vi "Dashboard Main.vi"() -> ()   [LabVIEW 2018]
uses:
  <vilib>/Rock Robotics/WPI/Camera/WPI_CameraSettings Read MJPG.ctl
  <vilib>/Rock Robotics/WPI/Camera/WPI_CameraImageSize.ctl
  <vilib>/Utility/miscctls.llb/LVPointTypeDef.ctl
  <vilib>/Utility/miscctls.llb/LVBoundsTypeDef.ctl
  <vilib>/Rock Robotics/Network Tables/NT Read Number.vi
  <vilib>/Rock Robotics/Network Tables/NT Write String.vi
  <vilib>/Rock Robotics/Network Tables/NT Write Number.vi
  <vilib>/Rock Robotics/WPI/Dashboard/WPI_DashboardLogging Global.vi
  <vilib>/Rock Robotics/Network Tables/NT Read Variant.vi
panel:
  out "Camera Perf":string
  out "Right Camera Perf":cluster{"Bandwidth (Mbps)":dbl, "FPS":dbl}
  out "NT Connection":bool
  in  "Driver Configuration":enum16{"James", "Ryan"}(ring)
  in  "Camera Settings Right":T1={"Frame Rate"=30, "Compression"=30, "Size"=1, "DB Camera Config"=FALSE} {"Frame Rate" scale=1.0..30.0; "Compression" scale=100.0..-1.0; "Size" items=["640x480", "320x240", "160x120"]}
  in  "Camera Name Right":string(combo)="No Camera Selection"
  in  "TCP":refnum<k5>
  in  "Rec Mode":enum32{"Stop", "Record", "Playback"}(radio)
  out "Robot IP":string
  out "Image Message":string="Timeout in Camera Communications"
  in  "Dashboard Tab":T2(tab)
  out "Pressure":u8(slide) scale=0.0..140.0
  out "Time":dbl
  out "Camera Image Right":T3(plugin-control)
  in  "Camera Settings":T4={"fps"=30, "compression"=30, "Image Size"=enum."320x240", "Config Shown"=FALSE}
  out "Endgame?":bool
  out "Stilts":bool
  out "Rhino":bool
  out "Floating":bool
  out "Carriage":bool
  out "Cascade":bool
  out "Errors":string
  out "Drive Base":bool
  out "Postmatch Pressure Log":dbl(graph)
  out "Mode":T6(ring)=enum."Auto Disabled"
  out "IMU":dbl
  out "Picture":picture
  in  "Autonomous Selector":T7(ring)
  out "Picture 2":picture
  out "Tree":string(tree)
  # "HW"
  # "Robot Health"
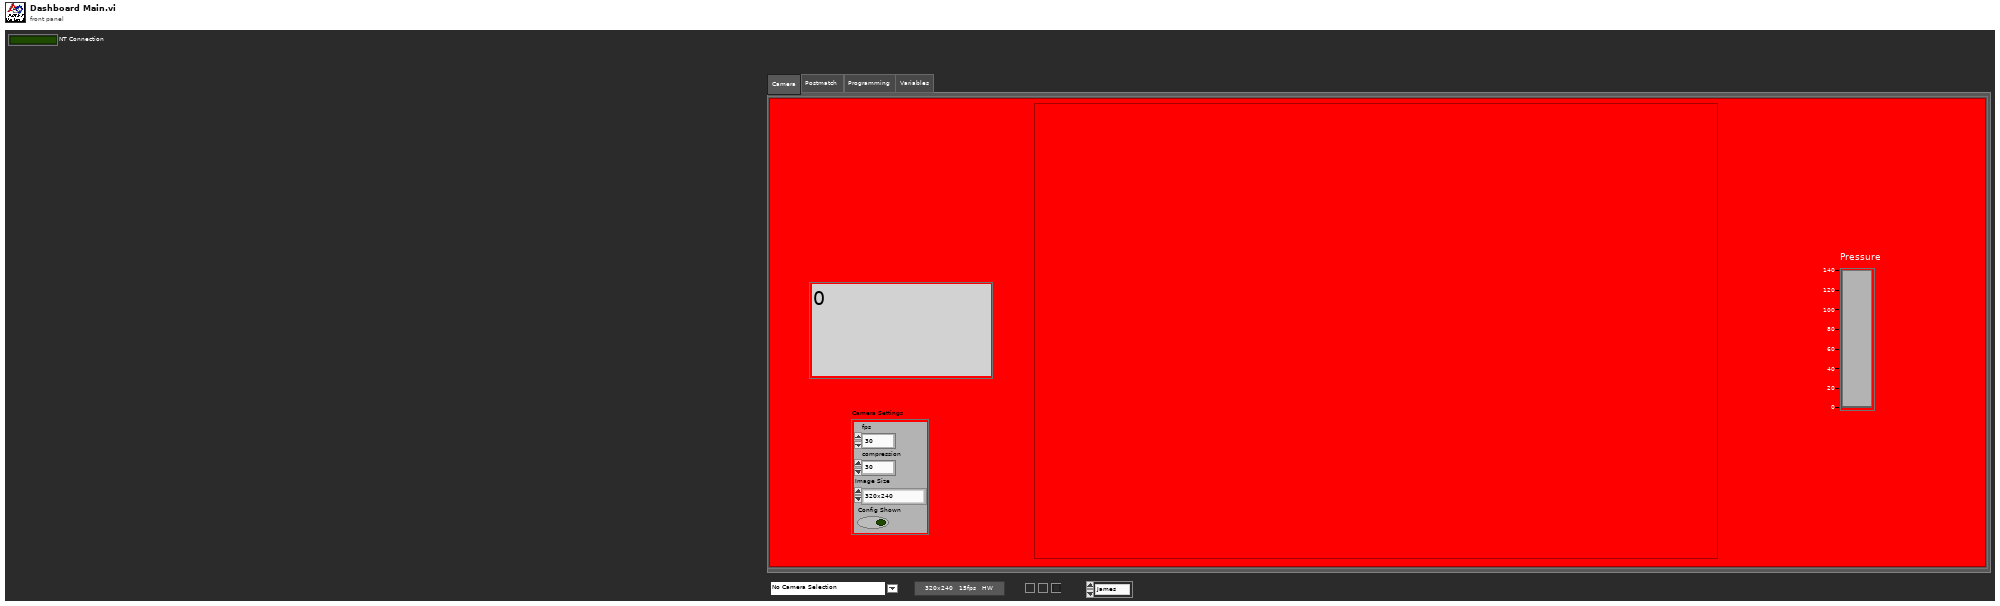
[diagram p1: front panel]
types:
  T1 = cluster{"Frame Rate":i32, "Compression":i32, "Size":u16, "DB Camera Config":bool}
  T2 = enum32{"Camera", "Postmatch", "Programming", "Variables"}
  T3 = typedef "IMAQ Image.ctl" = refnum<image>
  T4 = typedef "WPI_CameraSettings Read MJPG.ctl" = cluster{"fps":i32, "compression":i32, "Image Size":T5, "Config Shown":bool}
  T5 = typedef "WPI_CameraImageSize.ctl" = enum16{"640x480", "320x240", "160x120", "Custom"}
  T6 = enum8{"Tele-Op Disabled", "Tele-Op Enabled", "Auto Disabled", "Auto Enabled", "Test Disabled", "Test Enabled", "Disconnected", "No Code", "E-Stop"}
  T7 = enum16{"Teleop", "Double Rocket L", "Double Rocket R", "Side Cargo L", "Side Cargo R", "Double Front L", "Double Front R"}
  T8 = typedef "LVBoundsTypeDef.ctl" = cluster{"Width":u32, "Height":u32}
  T9 = typedef "LVPointTypeDef.ctl" = cluster{"Horizontal":i16, "Vertical":i16}
  T10 = cluster{"Save Path":path, "Interval (s)":dbl, "Keep":i32}
  T11 = enum32{"Drive", "Camera", "Basic", "Custom", "Test", "Commands", "Checklist", "Variables"}
  T12 = typedef "Image Type" = u32
  T13 = cluster{"IDs":cluster{"RPC field ID":u16, "Unique ID":u16}, "String":string}
  T14 = enum8{"Enabled", "Disabled", "Disabled and Grayed Out"}
  T15 = cluster{"Error Strings":string, "Disable Counts":cluster{u16, u16}, "Rail Faults":cluster{u16, u16, u16}, "Robot IP":string, "DB Mode":u8, "Event Info":cluster{"Name":string, "Type":u8, "Number":u16, "Replay":u8}}
  T16 = cluster{"Storage":cluster{"Disk Free":u64, "RAM Block":u32, "RAM free":u32}, "CPU Utilization":cluster{"CPU % ISR":sgl, "CPU % Time Crit":sgl, "CPU % Timed Str":sgl, "CPU % High":sgl, "CPU % Above":sgl, "CPU % Normal":sgl, "CPU % Low":sgl}, "CAN":cluster{"% Bus Utilization":sgl, "Bus Off Cnt":u32, "TX_FIFO Full Cnt":u32, "Receive Error Cnt":u8, "Transmit Error Cnt":u8}, "HID":cluster{"HID Outputs":u32, "Rumble Low":u16, "Rumble High":u16}[]}
  T17 = cluster{"Status bits":cluster{"Test Mode":bool, "Autonomous":bool, "Enabled":bool, "Code Start":bool, "Brownout":bool, "Reserved 2":bool, "Reserved 3":bool, "E-Stop":bool}, "Code Trace":cluster{"Disabled":bool, "TeleOp":bool, "Auto":bool, "Test":bool}, "Controller Type":enum16{"unknown", "cRIO", "roboRio"}, "Code?":enum16{"unknown", "noCode", "code"}, "Battery V":dbl}
  T18 = cluster{"Control Bits":cluster{"TestMode":bool, "Autonomous":bool, "Enabled":bool, "FMS Present":bool, bool, bool, bool, "E-Stop":bool}, "Team Station ":u8, "Countdown":sgl, "Joystick Values":cluster{"Axes":dbl[], "Buttons":bool[], "POVs":i16[]}[]}
  T19 = cluster{"Axes":dbl[], "Buttons":bool[], "POVs":i16[]}[]
  T20 = cluster{"Axes":dbl[], "Buttons":bool[], "POVs":i16[]}
  T21 = cluster{"Global Rectangle":i32[], "Contours":cluster{"Contour Type":u32, "ROI Type":u32, "Points":i32[]}[]}
  T22 = cluster{"Camera Name Right":string, string, "Saved DB Images Info":cluster{"Save Path":path, "Interval (s)":dbl, "Keep":i32}}
  T23 = cluster{"Operation":enum16{"Update", "Clear"}, "Color Box":u32}[]
  T24 = cluster{"Image Size":bool, "Image Type":bool, "Pixel Value":bool, "ROI Information":bool, "Zoom Factor":bool}
  T25 = cluster{"Shift":bool, "Ctrl":bool, "Alt":bool, "Cmd":bool, "Opt":bool}
  T26 = cluster{"Segment Name":string, "Type":enum16{"Accel Straight", "Const Straight", "Blend", "Circle"}, "Traj Pos Points":cluster{"x":dbl, "y":dbl, "th":dbl}[], "Traj Vel Points":cluster{"V":dbl, "th":dbl}[], "Accel Index":i32, "Decel Index":i32}[]
  T27 = cluster{"Index":i32, "Pt Test Results":enum16{"Miss", "Rect Hit", "Arrow Hit"}}
  T28 = cluster{"Points":cluster{"x":dbl, "y":dbl, "th":dbl}[], "Trajectory Data":cluster{"Segment Name":string, "Type":enum16{"Accel Straight", "Const Straight", "Blend", "Circle"}, "Traj Pos Points":cluster{"x":dbl, "y":dbl, "th":dbl}[], "Traj Vel Points":cluster{"V":dbl, "th":dbl}[], "Accel Index":i32, "Decel Index":i32}[]}
  T29 = cluster{"Points":cluster{"x":dbl, "y":dbl, "th":dbl}[], "Trajectory Data":cluster{"Segment Name":string, "Type":enum16{"Accel Straight", "Const Straight", "Blend", "Circle"}, "Traj Pos Points":cluster{"x":dbl, "y":dbl, "th":dbl}[], "Traj Vel Points":cluster{"V":dbl, "th":dbl}[], "Accel Index":i32, "Decel Index":i32}[]}[]
  T30 = cluster{"Horizontal":dbl, "Vertical":dbl, "th":dbl}
  T31 = typedef "imagedata.ctl" = cluster{"image type":i32, "image depth":i32, "image":u8[], "mask":u8[], "colors":u32[], "Rectangle":cluster{"left":i16, "top":i16, "right":i16, "bottom":i16}}
  T32 = typedef "LVRectTypeDef.ctl" = cluster{"Left":i16, "Top":i16, "Right":i16, "Bottom":i16}
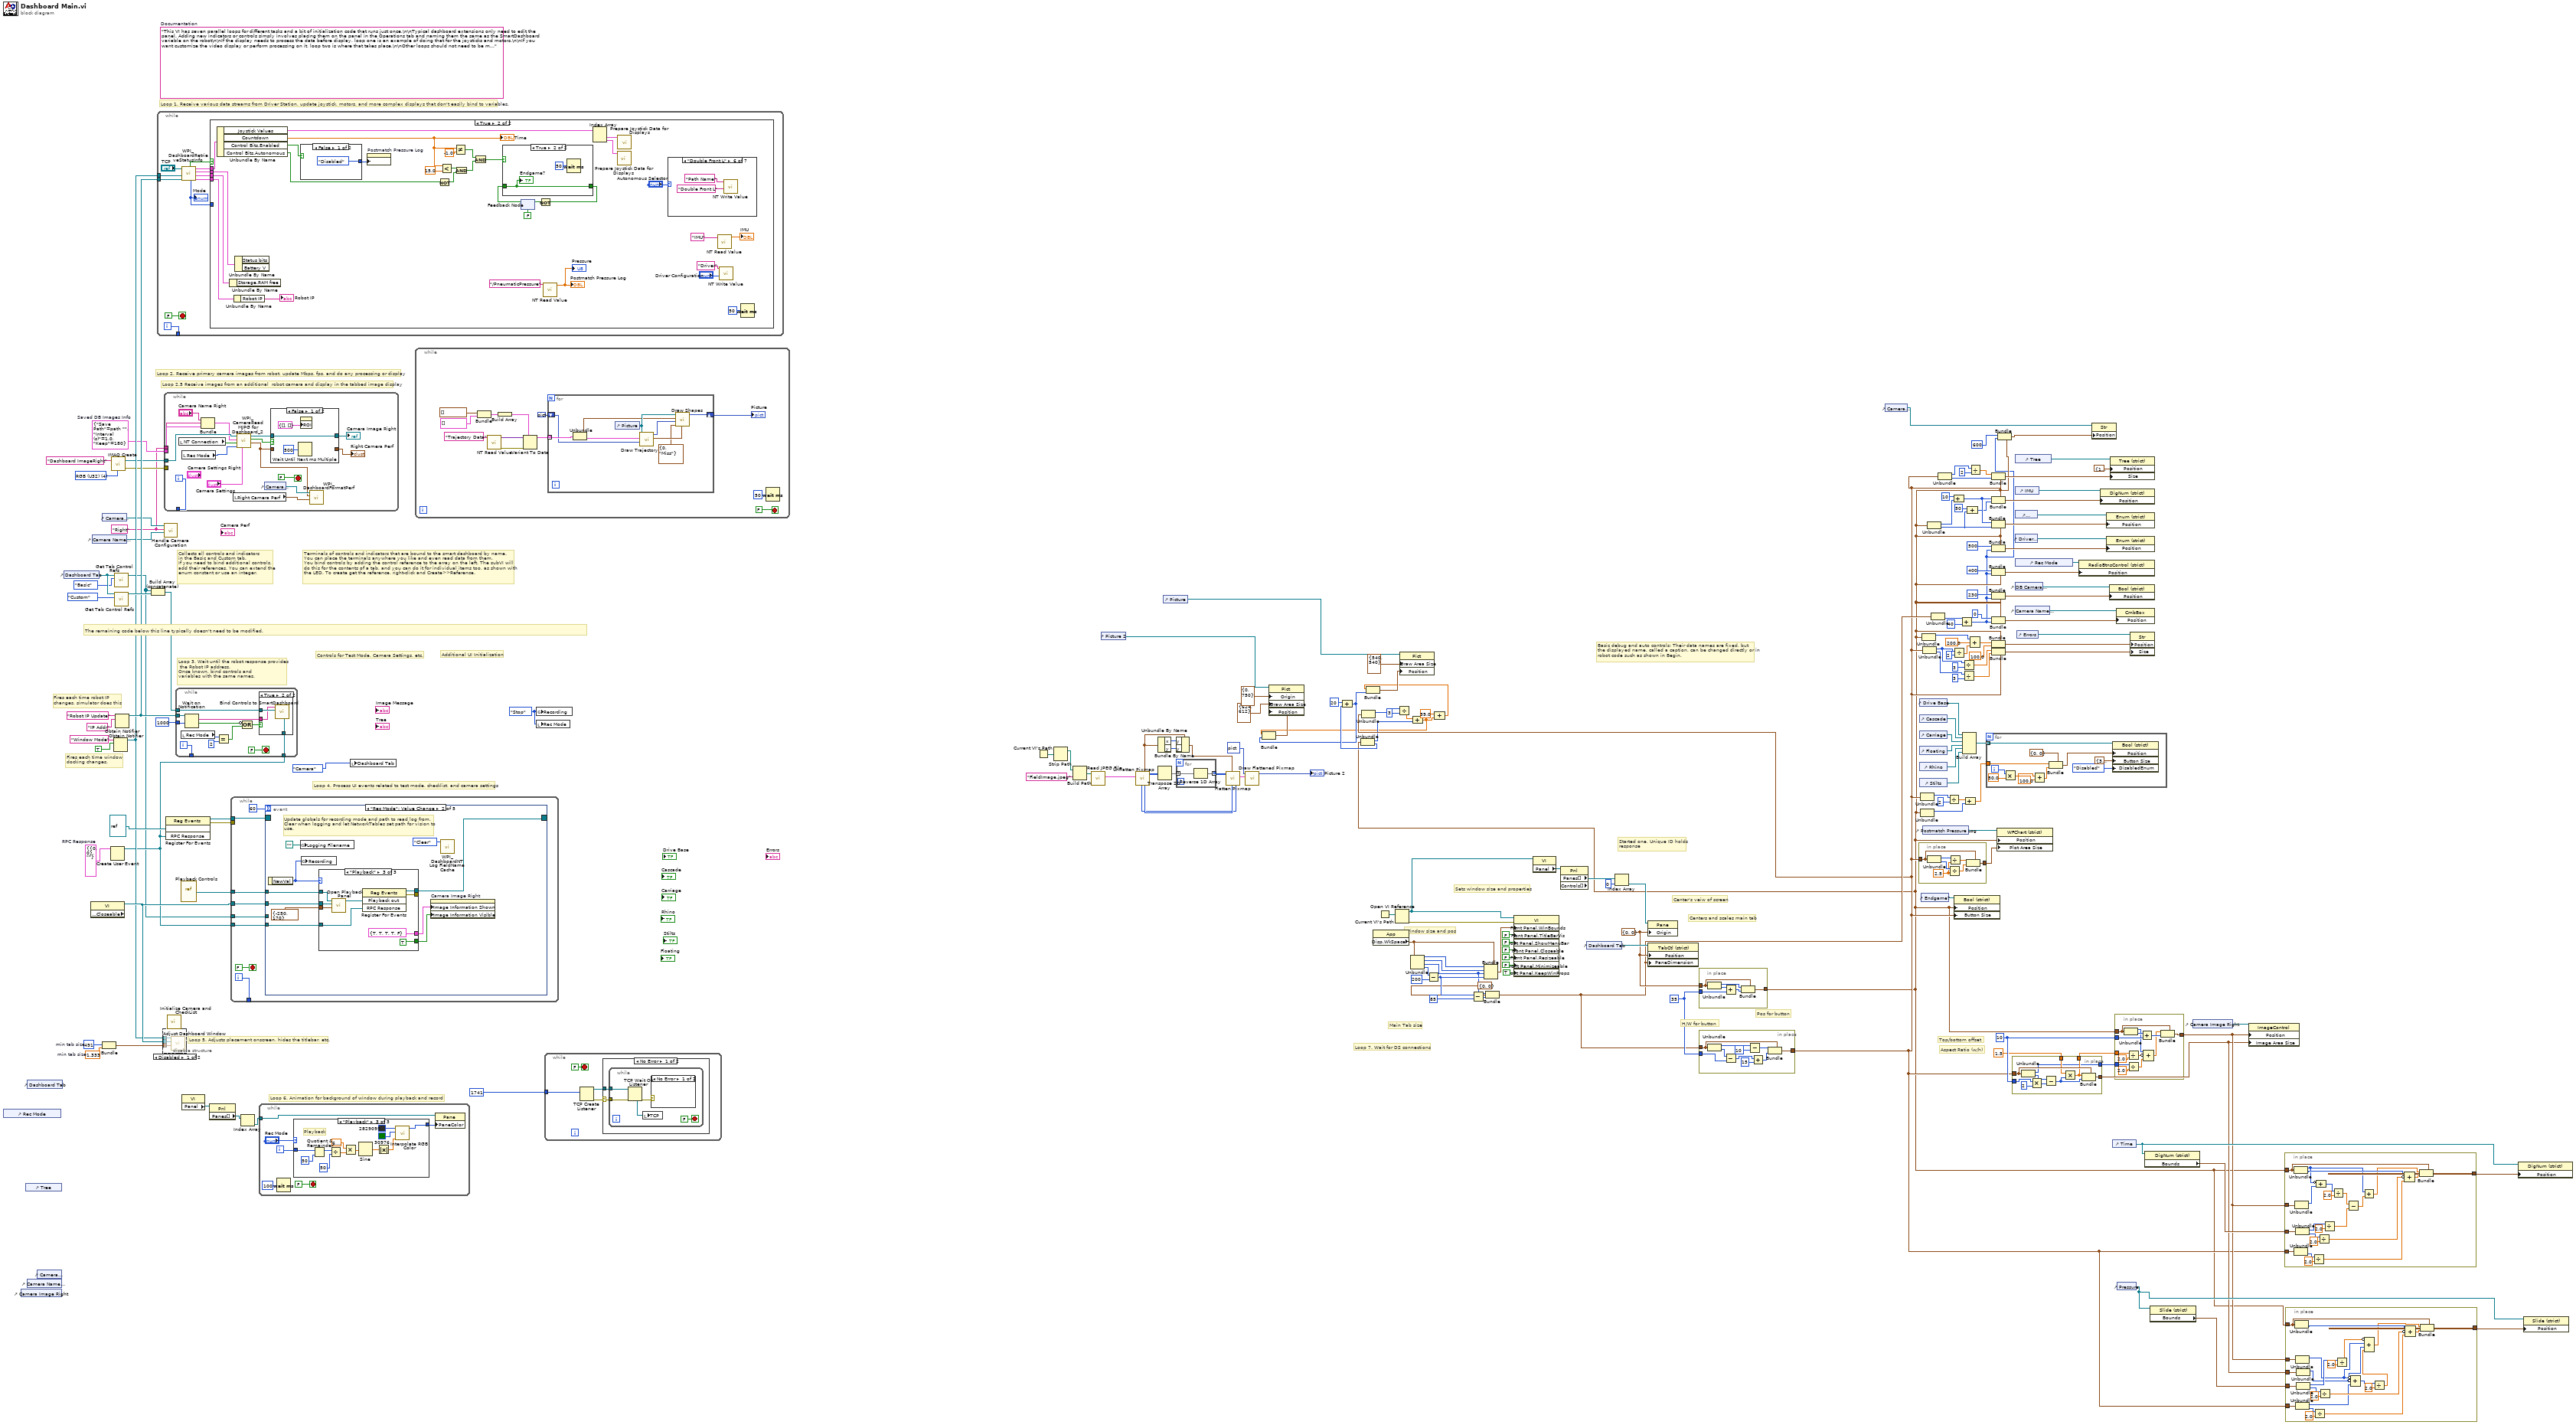
[diagram p0: block diagram]
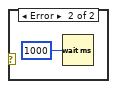
[diagram p4: hidden frame]
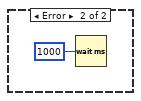
[diagram p5: hidden frame]
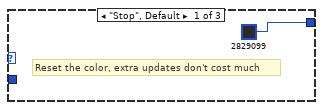
[diagram p6: hidden frame]
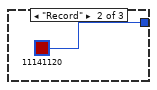
[diagram p7: hidden frame]
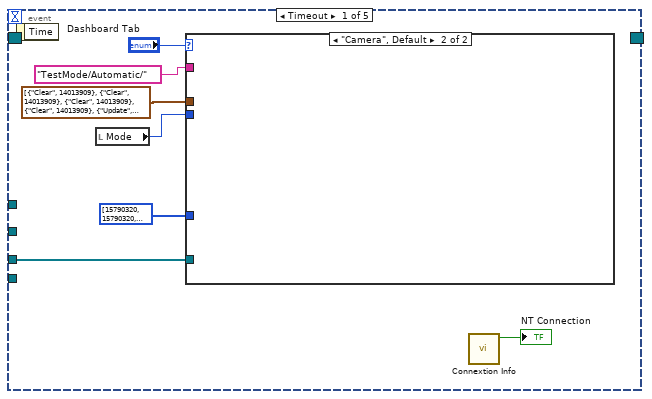
[diagram p9: hidden frame]
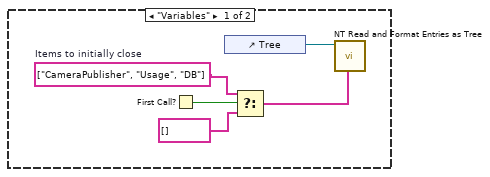
[diagram p10: hidden frame]
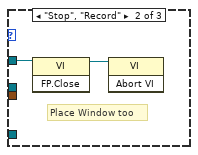
[diagram p12: hidden frame]
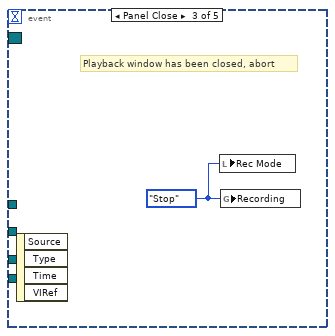
[diagram p13: hidden frame]
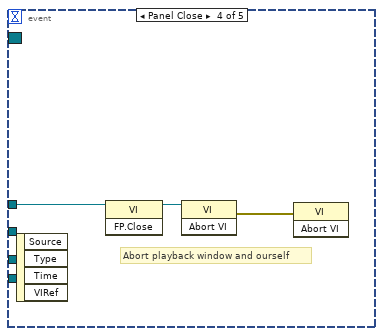
[diagram p14: hidden frame]
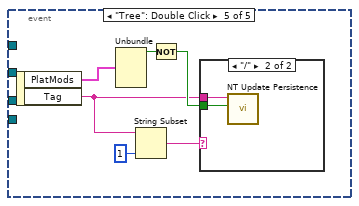
[diagram p15: hidden frame]
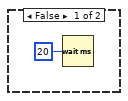
[diagram p17: hidden frame]
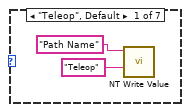
[diagram p18: hidden frame]
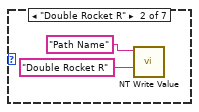
[diagram p19: hidden frame]
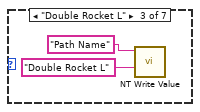
[diagram p20: hidden frame]
diagram:
  w114 = i16 10 ("y")
  w116 = 35 ("y")
  w117 = cluster{"X":i32, "Y":i32} {"X"=0, "Y"=0}
  w145 = T10 {"Save Path"=path "", "Interval (s)"=1.0, "Keep"=180}  # Saved DB Images Info
  w144 = "Right"
  w152 = T12 4 items=["Grayscale (U8)", "Grayscale (I16)", "Grayscale (SGL)", "Complex (CSG)", "RGB (U32)", "HSL (U32)", "RGB (U64)"] ("Image Type")
  w156 = T13 {"IDs"={"RPC field ID"=0, "Unique ID"=0}, "String"=""}  # RPC Response
  w162 = 491  # min tab size
  w161 = 1.333  # min tab size
  w167 = enum32{"Stop", "Record", "Playback"}."Stop" ("Rec Mode")
  (unwired) "This VI has seven parallel loops for different tasks and a bit of initialization code that runs just once.\n\nTypical dashboard extensions only need to edit the panel. Adding new indicators or controls simply involves placing them on the panel in the Operations tab and naming them the same as the SmartDashboard variable on the robot\n\nIf the display needs to process the data before display, loop one is an example of doing that for the joysticks and motors.\n\nIf you want customize the video display or perform processing on it, loop two is where that takes place.\n\nOther loops should not need to be modified. They are pretty standard, and document the task they perform."  # Documentation
  # "Aspect Ratio (w/h)"
  # "Top/bottom offset"
  # "H/W for button"
  # "Pos for button"
  # "Centers and scales main tab"
  # "Center's veiw of screen"
  # "Main Tab size"
  # "Window size and pos"
  # "Sets window size and properties"
  # "Loop 2.5 Receive images from an additional  robot camera and display in the tabbed image display"
  # "Started one, Unique ID holds\nresponse"
  # "Loop 7. Wait for DS connections"
  # "Basic debug and auto controls: Their data names are fixed, but\nthe displayed name, called a caption, can be changed directly or in\nrobot code such as shown in Begin."
  # "Controls for Test Mode, Camera Settings, etc."
  # "Additional UI Initialization"
  # "Loop 6. Animation for background of window during playback and record"
  # "Fires each time robot IP\nchanges, simulator does this"
  # "Fires each time window\ndocking changes."
  # "Collects all controls and indicators\nin the Basic and Custom tab.\nIf you need to bind additional controls,\nadd their references. You can extend the\nenum constant or use an integer."
  # "The remaining code below this line typically doesn't need to be modified."
  # "Loop 4. Process UI events related to test mode, checklist, and camera settings"
  # "Terminals of controls and indicators that are bound to the smart dashboard by name.\nYou can place the terminals anywhere you like and even read data from them.\nYou bind controls by adding the control reference to the array on the left. The subVI will\ndo this for the contents of a tab, and you can do it for individual items too, as shown with\nthe LED. To create get the reference, right-click and Create>>Reference."
  # "Loop 3. Wait until the robot response provides\n the Robot IP address.\nOnce known, bind controls and\nvariables with the same names."
  # "Loop 5. Adjusts placement onscreen, hides the titlebar, etc."
  # "Loop 1. Receive various data streams from Driver Station, update joystick, motors, and more complex displays that don't easily bind to variables."
  # "Loop 2. Receive primary camera images from robot, update Mbps, fps, and do any processing or display"
  n1 = control-ref of="Rec Mode"() -> ()  [unwired: 1 out]
  n2 = control-ref of="Camera Image Right"() -> ()  [unwired: 1 out]
  n3 = control-ref of="Tree"() -> ()  [unwired: 1 out]
  n4 = control-ref of="Dashboard Tab"() -> ()  [unwired: 1 out]
  n5 = control-ref of="Camera Name Right"() -> ()  [unwired: 1 out]
  n6 = control-ref of="Camera Settings Right"() -> ()  [unwired: 1 out]
  n7 = control-ref of="Dashboard Tab"() -> (w165:refnum<vi>)
  n8 = property class="VI" props=["Front Panel.Closeable"]() -> (reference out=w166:refnum<vi>)  [unwired: 2 in, 2 out]
  n9 = control-ref of="Camera Name Right"() -> (w148:refnum<vi>)
  n10 = control-ref of="Camera Settings Right"() -> (w149:refnum<vi>)
  n11 = Bundle("min tab size"=w162, "min tab size"=w161) -> (w160:cluster{"min tab size":i32, "min tab size":dbl})  [unwired: 1 in]
  n12 = Create User Event(user event datatype=w156) -> (user event=w155:refnum<user-event>)  [unwired: 1 in, 1 out]
  n13 = call "IMAQ Create"("Image Name"="Dashboard ImageRight", "Image Type"=w152) -> ("New Image"=w151:T3, "error out"=w150:errorcluster)  [unwired: 2 in, 1 out]
  n14 = Obtain Notifier(name (unnamed)="Window Mode", notification data type=TRUE) -> (notifier out=w158:refnum<notifier>)  [unwired: 2 in, 2 out]
  n15 = call <vilib>:"Get Tab Control Refs.vi"("Page Index"=T11."Basic" ("Dashboard Tab"), "TabControl in"=w165) -> ("ControlsOnPage"=w154:refnum<vi>[])  [unwired: 9 in]
  n16 = call <vilib>:"Get Tab Control Refs.vi"("Page Index"=T11."Custom" ("Dashboard Tab"), "TabControl in"=w165) -> ("ControlsOnPage"=w164:refnum<vi>[])  [unwired: 9 in]
  n17 = Obtain Notifier(name (unnamed)="Robot IP Update", notification data type="IP Addr" ("name (unnamed)")) -> (notifier out=w159:refnum<notifier>)  [unwired: 2 in, 2 out]
  n18 = Build Array (concatenate)(w154, w164) -> (w163:refnum<vi>[])
  n19 = while {
    tunnel: [w189] -> _
    tunnel: w159 -> [w183]
    tunnel: w158 -> [w180]
    i -> [w189]
    stop <- FALSE stop-if-true
    n20 = call <vilib>:"WPI_DashboardRetrieveStatusInfo.vi"("Binding Refnum"=w183, "Window Mode Notifier"=w180, "TCP Cnx"="TCP") -> ("Power and Errors"=w184:T15, "Robot Metrics"=w187:T16, "Status Info"=w188:T17, "Control Info"=w185:T18, "Robot Mode"=w182:T6, "Process?"=w186:bool)  [unwired: 3 in]
    "Mode" <- w182
    n21 = case shown="True" w186 {
      tunnel: w188 -> [_ w222]
      tunnel: w187 -> [_ w221]
      tunnel: w185 -> [_ w220]
      tunnel: w184 -> [_ w219]
      tunnel: w182 -> [_ _]
      frame False {
        n22 = Wait (ms)(milliseconds to wait=u32 20) -> ()  [unwired: 1 out]
      }
      frame True {
        n23 = Unbundle By Name(w220) -> ("Joystick Values"=w218:T19, "Countdown"=w200:sgl, "Control Bits.Enabled"=w213:bool, "Control Bits.Autonomous"=w211:bool)
        "Time" <- w200
        n24 = Unbundle By Name(w221) -> ()  [unwired: 1 out]
        n25 = Unbundle By Name(w219) -> ("Robot IP"=→"Robot IP":string)
        n26 = Unbundle By Name(w222) -> ()  [unwired: 2 out]
        n27 = case shown="False" w213 {
          tunnel: [T14."Disabled" ("Disabled") T14."Enabled" ("Disabled")] -> w212
          frame False {
          }
          frame True {
          }
        }
        n28 = property on="Postmatch Pressure Log" class="WFChart (strict)"("DisabledEnum"=w212) -> ()  [unwired: 2 in, 2 out]
        n29 = Not(x=w211) -> (.not. x?=w210:bool)
        n30 = Less?(x=w200, y=sgl 15.0) -> (x < y?=w209:bool)
        n31 = Not Equal?(x=w200, y=sgl -1.0) -> (x != y?=w202:bool)
        n32 = And(x=w209, y=w210) -> (x .and. y?=w201:bool)
        n33 = And(x=w202, y=w201) -> (x .and. y?=w198:bool)
        n34 = feedback #1(FALSE ("Endgame?")) -> (w205:bool)
        n35 = Not(x=w205) -> (.not. x?=w204:bool)
        n36 = case shown="True" w198 {
          tunnel: [w237 w239] -> w206
          tunnel: w204 -> [w237 w239]
          frame False {
          }
          frame True {
            n37 = Wait (ms)(milliseconds to wait=u32 50) -> ()  [unwired: 1 out]
            "Endgame?" <- w239
          }
        }
        n38 = feedback-in #1(w206) -> ()
        n39 = call-poly <vilib>:"NT Read Value.vi"("Name"="/PneumaticPressure") -> ("Numeric"=→"Postmatch Pressure Log" →"Pressure":dbl)  [unwired: 9 in, 1 out]
        n40 = Index Array(array=w218) -> (element #1=w217:T20, element #2=w216:T20)  [unwired: 2 in]
        n41 = call "Prepare Joystick Data for Displays.vi"("Joystick Values"=w216) -> ()  [unwired: 8 in, 3 out]
        n42 = call "Prepare Joystick Data for Displays.vi"("Joystick Values"=w217) -> ()  [unwired: 8 in, 3 out]
        n43 = case shown="\"Double Front L\"" "Autonomous Selector" {
          frame "Teleop", Default {
            n44 = call-poly <vilib>:"NT Write Value.vi"("String"="Teleop" ("Name"), "Name"="Path Name") -> ()  [unwired: 9 in, 1 out]
          }
          frame "Double Rocket R" {
            n45 = call-poly <vilib>:"NT Write Value.vi"("String"="Double Rocket R" ("Name"), "Name"="Path Name") -> ()  [unwired: 9 in, 1 out]
          }
          frame "Double Rocket L" {
            n46 = call-poly <vilib>:"NT Write Value.vi"("String"="Double Rocket L" ("Name"), "Name"="Path Name") -> ()  [unwired: 9 in, 1 out]
          }
          frame "Side Cargo L" {
            n47 = call-poly <vilib>:"NT Write Value.vi"("String"="Side Cargo L" ("Name"), "Name"="Path Name") -> ()  [unwired: 9 in, 1 out]
          }
          frame "Side Cargo R" {
            n48 = call-poly <vilib>:"NT Write Value.vi"("String"="Side Cargo R" ("Name"), "Name"="Path Name") -> ()  [unwired: 9 in, 1 out]
          }
          frame "Double Front L" {
            n49 = call-poly <vilib>:"NT Write Value.vi"("String"="Double Front L" ("Name"), "Name"="Path Name") -> ()  [unwired: 9 in, 1 out]
          }
          frame "Double Front R" {
            n50 = call-poly <vilib>:"NT Write Value.vi"("String"="Double Front R" ("Name"), "Name"="Path Name") -> ()  [unwired: 9 in, 1 out]
          }
        }
        n51 = call-poly <vilib>:"NT Read Value.vi"("Name"="IMU") -> ("Numeric"=→"IMU":dbl)  [unwired: 9 in, 1 out]
        n52 = call-poly <vilib>:"NT Write Value.vi"("Numeric"="Driver Configuration", "Name"="Driver") -> ()  [unwired: 9 in, 1 out]
        n53 = Wait (ms)(milliseconds to wait=u32 50) -> ()  [unwired: 1 out]
      }
    }
  }
  n54 = disable-structure shown="Disabled" {
    disable-tunnel: w166 -> [w244 _]
    disable-tunnel: w160 -> [w243 _]
    disable-tunnel: w158 -> [w242 _]
    frame Disabled {
      n55 = call "Adjust Dashboard Window.vi"("Size Constraints"=w243, "VI"=w244, "WIn Mode"=w242) -> ()  [unwired: 9 in]
    }
    frame Enabled {
    }
  }
  n56 = call "Handle Camera Configuration.vi"("CameraNameRef"=w148, "Display Name"=w144, "ClusterRef"=w149) -> ()  [unwired: 9 in]
  n57 = while {
    tunnel: w151 -> [w261]
    tunnel: w150 -> [_]
    tunnel: [w257] -> _
    tunnel: w145 -> [w254]
    tunnel: w144 -> [w251]
    i -> [w257]
    stop <- FALSE stop-if-true
    n58 = local read "NT Connection"() -> (w250:bool)
    n59 = local read "Rec Mode"() -> (w260:enum32{"Stop", "Record", "Playback"})
    n60 = Bundle("Camera Name Right"="Camera Name Right", w251, "Saved DB Images Info"=w254) -> (w253:T22)  [unwired: 1 in]
    n61 = local read "Right Camera Perf"() -> (w247:cluster{"Bandwidth (Mbps)":dbl, "FPS":dbl})
    n62 = call <vilib>:"WPI_CameraRead MJPG for Dashboard_2.vi"("Camera Settings"="Camera Settings", "Rec Mode"=w260, "NT Connection"=w250, "Capture Info"=w253, "Image in"=w261) -> ("perf info"=w246:cluster{"Bandwidth (Mbps)":dbl, "fps":dbl}, "Active"=w256:bool, "Image\\ out"=w259:T3)  [unwired: 4 in]
    n63 = control-ref of="Camera Perf"() -> (w248:refnum<vi>)
    n64 = case shown="False" w256 {
      tunnel: w259 -> [w263 w266]
      tunnel: [w263 w266] -> w255
      tunnel: [_ w265] -> w249
      tunnel: w246 -> [_ w265]
      frame False {
        n65 = Wait Until Next ms Multiple(millisecond multiple=u32 500) -> ()  [unwired: 1 out]
        n66 = property on="Camera Image Right" class="ImageControl"("ROI"=T21 {"Global Rectangle"=[], "Contours"=[]}) -> ()  [unwired: 2 in, 2 out]
      }
      frame True {
      }
    }
    "Camera Image Right" <- w255
    "Right Camera Perf" <- w249
    n67 = call <vilib>:"WPI_DashboardFormatPerf.vi"("Right Camera Perf"=w247, "Performance"=w246, "String in"=w248) -> ()  [unwired: 9 in]
  }
  n68 = register-events(refnum<vi> refnum, w155) -> (reference out=w171:refnum<event-registration>, error out=w170:errorcluster)  [unwired: 2 in]
  n69 = call "Initialize Camera and CheckList.vi"() -> ()  [unwired: 12 in]
  n70 = while {
    tunnel: w163 -> [w278]
    tunnel: w159 -> [w276]
    tunnel: [w274] -> _
    tunnel: u32 1000 ("milliseconds to wait") -> [w273]
    tunnel: w155 -> [w267]
    i -> [w274]
    stop <- FALSE stop-if-true
    n71 = local read "Rec Mode"() -> (w269:enum32{"Stop", "Record", "Playback"})
    n72 = Wait on Notification(notifier=w276, timeout in ms (-1)=w273) -> (notification=w275:string, timed out?=w271:bool)  [unwired: 2 in, 2 out]
    n73 = Equal?(x=w269, y=u16 2 ("Rec Mode")) -> (x = y?=w270:bool)
    n74 = Compound Arithmetic op=OR(invert w271, w270) -> (w272:bool)
    n75 = case shown="True" w272 {
      tunnel: w278 -> [_ w281]
      tunnel: w275 -> [_ w280]
      tunnel: w267 -> [_ w279]
      frame False {
      }
      frame True {
        n76 = call <vilib>:"Bind Controls to SmartDashboard.vi"("RPC ref"=w279, "Bound Control Refs"=w281, "Server IP Address"=w280) -> ()  [unwired: 9 in]
      }
    }
  }
  n77 = vi-ref "Playback Controls.vi"() -> (w172:refnum<vi>)
  n78 = property class="VI"() -> ("Panel"=w174:refnum<vi>)  [unwired: 2 in, 2 out]
  n79 = property class="Pnl"(reference=w174) -> ("Panes[]"=w175:refnum<vi>[])  [unwired: 1 in, 2 out]
  n80 = while {
    tunnel: [w287] -> _
    tunnel: w172 -> [w286]
    tunnel: w171 -> [w285]
    tunnel: w170 -> [_]
    tunnel: w166 -> [w284]
    tunnel: w155 -> [w283]
    tunnel: w154 -> [w282]
    i -> [w287]
    stop <- FALSE stop-if-true
    n81 = event shown="[1] \"Rec Mode\": Value Change" {
      selector: w285 -> [_ _ _ _ _]
      dyn-events: [_ w308 _ _ _] -> _
      timeout: u32 60 ("milliseconds to wait") -> [_ _ _ _ _]
      tunnel: w286 -> [_ w310 _ w326 _]
      tunnel: w284 -> [_ w306 _ _ _]
      tunnel: w283 -> [_ w304 _ _ _]
      tunnel: w282 -> [w291 _ _ _ _]
      event Timeout {
        n82 = event-data() -> ()  [unwired: 1 in, 1 out]
        n83 = local read "Mode"() -> (w294:T6)
        n84 = case shown="\"Camera\", Default" "Dashboard Tab" {
          tunnel: "TestMode/Automatic/" ("Name Pattern") -> [_ _]
          tunnel: T23 [{"Operation"=enum."Clear", "Color Box"=14013909}, {"Operation"=enum."Clear", "Color Box"=14013909}, {"Operation"=enum."Clear", "Color Box"=14013909}, {"Operation"=enum."Clear", "Color Box"=14013909}, {"Operation"=enum."Update", "Color Box"=14013909}, {"Operation"=enum."Update", "Color Box"=16777215}, {"Operation"=enum."Clear", "Color Box"=14013909}, {"Operation"=enum."Clear", "Color Box"=14013909}, {"Operation"=enum."Clear", "Color Box"=14013909}] -> [_ _]
          tunnel: w294 -> [_ _]
          tunnel: u32[] [15790320, 15790320, 15790320, 15790320, 16777215, 16777215, 15790320, 15790320, 15790320] -> [_ _]
          tunnel: w291 -> [_ _]
          frame "Variables" {
            w299 = string[] ["CameraPublisher", "Usage", "DB"]  # Items to initially close
            n85 = First Call?() -> (First Call?: T/F=w300:bool)
            n86 = control-ref of="Tree"() -> (w301:refnum<vi>)
            n87 = Select(t=w299, s=w300, f=string[] []) -> (s? t:f=w297:string[])
            n88 = call <vilib>:"NT Read and Format Entries as Tree.vi"("Tags to  Close"=w297, "Tree Refnum"=w301) -> ()  [unwired: 8 in, 2 out]
          }
          frame "Camera", Default {
          }
        }
        n89 = call <vilib>:"Connextion Info.vi"() -> ("Connected"=→"NT Connection":bool)  [unwired: 10 in, 1 out]
      }
      event "Rec Mode": Value Change {
        # "Update globals for recording mode and path to read log from.\nClear when logging and let NetworkTables set path for vision to\nuse."
        n90 = event-data() -> ("NewVal"=w311:enum32{"Stop", "Record", "Playback"})  [unwired: 1 in]
        n91 = global write "WPI_DashboardLogging Global.vi" "Logging Filename"(path "") -> ()
        n92 = global write "WPI_DashboardLogging Global.vi" "Recording"(w311) -> ()
        n93 = case shown="\"Playback\"" w311 {
          tunnel: w310 -> [_ w313 w322]
          tunnel: [_ _ w321] -> w308
          tunnel: [_ _ w320] -> _
          tunnel: w306 -> [_ _ w318]
          tunnel: cluster{i32, i32} {-250, 170} -> [_ _ w317]
          tunnel: [_ _ T24 {"Image Size"=TRUE, "Image Type"=TRUE, "Pixel Value"=TRUE, "ROI Information"=TRUE, "Zoom Factor"=FALSE} ("Image Information Shown:All Elements")] -> w302
          tunnel: [_ _ TRUE ("Zoom Factor")] -> w303
          tunnel: w304 -> [_ _ w314]
          frame Default {
          }
          frame "Stop", "Record" {
            # "Place Window too"
            n94 = invoke class="VI" method="FP.Close"(reference=w313) -> (reference out=w312:refnum<vi>)  [unwired: 2 in, 2 out]
            n95 = invoke class="VI" method="Abort VI"(reference=w312) -> ()  [unwired: 2 in, 3 out]
          }
          frame "Playback" {
            n96 = call "Open Playback Panel.vi"("Offset"=w317, "DB VI Ref"=w318, "Playback in"=w322) -> ("Playback out"=w319:refnum<vi>)  [unwired: 8 in]
            n97 = register-events(w319, w314) -> (reference out=w321:refnum<event-registration>, error out=w320:errorcluster)  [unwired: 2 in]
          }
        }
        n98 = property on="Camera Image Right" class="ImageControl"("Image Information Shown"=w302, "Image Information Visible"=w303) -> ()  [unwired: 2 in, 2 out]
        n99 = call <vilib>:"WPI_DashboardNT Log FieldName Cache.vi"("Operation"=enum16{"Lookup/Add", "Index", "Clear"}."Clear") -> ()  [unwired: 8 in, 3 out]
      }
      event Panel Close {
        w323 = enum32{"Stop", "Record", "Playback"}."Stop" ("Rec Mode")
        # "Playback window has been closed, abort"
        n100 = event-data() -> ()  [unwired: 1 in, 4 out]
        n101 = local write "Rec Mode"(w323) -> ()
        n102 = global write "WPI_DashboardLogging Global.vi" "Recording"(w323) -> ()
      }
      event Panel Close {
        # "Abort playback window and ourself"
        n103 = event-data() -> ()  [unwired: 1 in, 4 out]
        n104 = invoke class="VI" method="FP.Close"(reference=w326) -> (reference out=w325:refnum<vi>)  [unwired: 2 in, 2 out]
        n105 = invoke class="VI" method="Abort VI"(reference=w325) -> (error out=w324:errorcluster)  [unwired: 2 in, 2 out]
        n106 = invoke class="VI" method="Abort VI"(error in=w324) -> ()  [unwired: 2 in, 3 out]
      }
      event "Tree": Double Click {
        n107 = event-data() -> ("PlatMods"=w332:T25, "Tag"=w329:string)  [unwired: 1 in]
        n108 = Unbundle(w332) -> ("Shift"=w331:bool)  [unwired: 4 out]
        n109 = String Subset(string=w329, length (rest)=1 ("length (rest)")) -> (substring=w328:string)  [unwired: 1 in]
        n110 = Not(x=w331) -> (.not. x?=w330:bool)
        n111 = case shown="\"/\"" w328 {
          tunnel: w329 -> [_ w334]
          tunnel: w330 -> [_ w333]
          frame Default {
          }
          frame "/" {
            n112 = call <vilib>:"NT Update Persistence.vi"("Persistence"=w333, "Name"=w334) -> ()  [unwired: 9 in, 1 out]
          }
        }
      }
    }
  }
  n113 = Index Array(array=w175) -> (element=w173:refnum<vi>)  [unwired: 1 in]
  n114 = while {
    tunnel: w173 -> [w336]
    i -> [w339]
    stop <- FALSE stop-if-true
    n115 = Wait (ms)(milliseconds to wait=u32 100) -> ()  [unwired: 1 out]
    n116 = case shown="\"Playback\"" "Rec Mode" {
      tunnel: w339 -> [_ _ w354]
      tunnel: [u32 2829099 ("Base Color") u32 11141120 ("Target Color") w343] -> w335
      frame "Stop", Default {
        # "Reset the color, extra updates don't cost much"
      }
      frame "Record" {
      }
      frame "Playback" {
        # "Playback"
        n117 = Quotient & Remainder(x=w354, y=u32 50 ("milliseconds to wait")) -> (x-y*floor(x/y)=w350:u32)  [unwired: 1 out]
        n118 = Divide(x=w350, y=u32 50 ("milliseconds to wait")) -> (x/y=w347:dbl)
        n119 = Multiply(x=6.283185307179586, y=w347) -> (x*y=w352:dbl)
        n120 = Sine(x=w352) -> (sin(x)=w351:dbl)
        n121 = Absolute Value(x=w351) -> (abs(x)=w344:dbl)
        n122 = call "Interpolate RGB Color.vi"("Proportion"=w344, "Target Color"=u32 30976, "Base Color"=u32 2829099) -> ("Result Color"=w343:u32)  [unwired: 8 in]
      }
    }
    n123 = property class="Pane"(reference=w336, "PaneColor"=w335) -> ()  [unwired: 1 in, 2 out]
  }
  n124 = local write "Dashboard Tab"(T2."Camera" ("Dashboard Tab")) -> ()
  n125 = while {
    stop <- FALSE stop-if-true
    n126 = Bundle("Points"=cluster{"x":dbl, "y":dbl, "th":dbl}[] [], "Trajectory Data"=T26 []) -> (w359:T28)  [unwired: 1 in]
    n127 = call-poly <vilib>:"NT Read Value.vi"("Name"="Trajectory Data") -> ("error out"=w363:errorcluster, "Variant"=w364:variant)  [unwired: 9 in]
    n128 = Build Array(w359) -> (w358:T29)
    n129 = Variant To Data(error in=w363, type=w358, Variant=w364) -> (data=w357:T29)  [unwired: 1 out]
    n130 = for {
      tunnel: w357 -> [w368] mode=indexing
      shift-right: [w373] -> w355
      shift-left: picture data[5B] ("new picture out") -> [w367]
      n131 = Unbundle(w368) -> ("Points"=w370:cluster{"x":dbl, "y":dbl, "th":dbl}[], "Trajectory Data"=w369:T26)
      n132 = control-ref of="Picture"() -> (w372:refnum<vi>)
      n133 = call "Draw Trajectory.vi"("new picture in"=w367, "Trajectory Data"=w369, "Picture in"=w372) -> ("Output Point"=w375:T30, "new picture"=w374:picture)  [unwired: 7 in]
      n134 = call "Draw Shapes.vi"("Output Point"=w375, "Results"=T27 {"Index"=0, "Pt Test Results"=enum."Miss"}, "new picture in"=w374, "Points"=w370, "Picture in"=w372) -> ("new picture out"=w373:picture)  [unwired: 6 in]
    }
    "Picture" <- w355
    n135 = Wait (ms)(milliseconds to wait=u32 50) -> ()  [unwired: 1 out]
  }
  n136 = global write "WPI_DashboardLogging Global.vi" "Recording"(w167) -> ()
  n137 = local write "Rec Mode"(w167) -> ()
  n138 = while {
    tunnel: u16 1741 ("timeout ms (25000)") -> [w377]
    stop <- FALSE stop-if-true
    n139 = TCP Create Listener(10:w377) -> (0:w376:errorcluster, 3:w378:refnum<k5>)  [unwired: 4 in, 1 out]
    n140 = case shown="No Error" w376 {
      selector: w376 -> [w380 _]
      tunnel: w378 -> [w381 _]
      frame No Error {
        n141 = while {
          tunnel: w381 -> [w384]
          tunnel: w380 -> [w383]
          stop <- FALSE stop-if-true
          n142 = TCP Wait On Listener(8:w383, 11:w384) -> (0:w385:errorcluster, 4:w386:refnum<k5>)  [unwired: 2 in, 3 out]
          n143 = local write "TCP"(w386) -> ()
          n144 = case shown="No Error" w385 {
            frame No Error {
            }
            frame Error {
              n145 = Wait (ms)(milliseconds to wait=u32 1000) -> ()  [unwired: 1 out]
            }
          }
        }
      }
      frame Error {
        n146 = Wait (ms)(milliseconds to wait=u32 1000) -> ()  [unwired: 1 out]
      }
    }
  }
  n147 = Current VI's Path() -> (path=w40:path)
  n148 = Strip Path(path=w40) -> (stripped path=w39:path)  [unwired: 1 out]
  n149 = Build Path(base path=w39, name or relative path="FieldImage.jpeg") -> (appended path=w37:path)
  n150 = call <vilib>:"Read JPEG File.vi"("path to JPEG file"=w37) -> ("image data"=w25:T31)  [unwired: 8 in, 2 out]
  n151 = control-ref of="Picture 2"() -> (w23:refnum<vi>)
  n152 = call <vilib>:"Unflatten Pixmap.vi"("image data"=w25) -> ("24-bit pixmap"=w33:u32[][], "colors"=w34:u32[], "top left"=w31:cluster{"x":i16, "y":i16}, "mask"=w26:u8[])  [unwired: 4 in, 3 out]
  n153 = Transpose 2D Array(2D array=w33) -> (transposed array=w27:u32[][])
  n154 = Unbundle By Name(w31) -> ("x"=w29:i16, "y"=w28:i16)
  n155 = control-ref of="Picture"() -> (w20:refnum<vi>)
  n156 = Bundle By Name(cluster=w31, "y"=w29, "y"=w28) -> (w30:cluster{"x":i16, "y":i16})
  n157 = for {
    tunnel: w27 -> [w390] mode=indexing
    tunnel: [w389] -> w32 mode=indexing
    n158 = Reverse 1D Array(array=w390) -> (reversed array=w389:u32[])
  }
  n159 = call <vilib>:"Flatten Pixmap.vi"("mask"=w26, "colors"=w34, "top left"=w30, "24-bit pixmap"=w32) -> ("image data"=w24:T31)  [unwired: 7 in]
  n160 = call <vilib>:"Draw Flattened Pixmap.vi"("image data"=w24, "picture"=picture data[5B]) -> ("new picture"=→"Picture 2":picture)  [unwired: 7 in]
  n161 = property class="App"() -> ("Disp.WkSpace"=w131:T32)  [unwired: 2 in, 2 out]
  n162 = Current VI's Path() -> (path=w142:path)
  n163 = Open VI Reference(vi path=w142) -> (vi reference=w128:refnum<vi>, error out=w141:errorcluster)  [unwired: 5 in]
  n164 = Unbundle(w131) -> ("Left"=w135:i16, "Top"=w134:i16, "Right"=w101:i16, "Bottom"=w133:i16)
  n165 = Subtract(x=w133, y=i16 200) -> (x-y=w122:i16)
  n166 = Subtract(x=w122, y=i16 85) -> (x-y=w121:i16)
  n167 = Bundle(cluster=w131, "Left"=w135, "Top"=w134, "Right"=w101, "Bottom"=w122) -> (w130:T32)
  n168 = Bundle(cluster=cluster{"Width":i16, "Height":i16} {"Width"=0, "Height"=0}, "Width"=w101, "Height"=w121) -> (w72:cluster{"Width":i16, "Height":i16})
  n169 = property class="VI"(reference=w128, error in=w141, "Front Panel.WinBounds"=w130, "Front Panel.TitleBarVis"=FALSE ("Front Panel Window:Title Bar Visible"), "Front Panel.ShowMenuBar"=FALSE ("Front Panel Window:Show Menu Bar"), "Front Panel.Closeable"=FALSE ("Front Panel Window:Closeable"), "Front Panel.Resizeable"=FALSE ("Front Panel Window:Resizable"), "Front Panel.Minimizeable"=FALSE ("Front Panel Window:Minimizable"), "Front Panel.KeepWinProps"=TRUE ("Front Panel Window:Keep Window Proportions")) -> ()  [unwired: 2 out]
  n170 = property class="VI"(reference=w128) -> ("Panel"=w127:refnum<vi>)  [unwired: 1 in, 2 out]
  n171 = property class="Pnl" props=["Panes[]", "Controls[]"](reference=w127) -> ("Panes[]"=w126:refnum<vi>[])  [unwired: 1 in, 3 out]
  n172 = control-ref of="Dashboard Tab"() -> (w123:refnum<vi>)
  n173 = Index Array(array=w126, index=0) -> (element=w124:refnum<vi>)
  n174 = property class="Pane"(reference=w124, "Origin"=w117) -> ()  [unwired: 1 in, 2 out]
  n175 = property class="TabCtl (strict)"(reference=w123, "Position"=w117, "PaneDimension"=w72) -> ()  [unwired: 1 in, 2 out]
  n176 = in-place {
    in-place-border: w117 -> [w396]
    in-place-border: [w395] -> w4
    in-place-border: w116 -> [w391]
    n177 = Unbundle(w396) -> ("X"=w394:i32, "Y"=w393:i32)
    n178 = Add(x=w393, y=w391) -> (x+y=w392:i32)
    n179 = Bundle(cluster=w396, "X"=w394, "Y"=w392) -> (w395:cluster{"X":i32, "Y":i32})
  }
  n180 = Unbundle(w4) -> ("X"=w17:i32, "Y"=w11:i32)
  n181 = Compound Arithmetic op=unknown(20 ("value"), w11) -> (w9:i32)
  n182 = in-place {
    in-place-border: w72 -> [w406]
    in-place-border: [w405] -> w18
    in-place-border: w116 -> [w402]
    n183 = Unbundle(w406) -> ("Width"=w399:i16, "Height"=w404:i16)
    n184 = Subtract(x=w404, y=w402) -> (x-y=w403:i32)
    n185 = Subtract(x=w399, y=i16 10) -> (x-y=w397:i16)
    n186 = Add(x=w403, y=15 ("x")) -> (x+y=w401:i32)
    n187 = Bundle(cluster=w406, "Width"=w397, "Height"=w401) -> (w405:cluster{"Width":i16, "Height":i16})
  }
  n188 = Unbundle(w18) -> ("Width"=w15:i16)  [unwired: 1 out]
  n189 = Divide(x=w15, y=i16 3) -> (x/y=w16:dbl)
  n190 = Compound Arithmetic op=ADD(w16, w17) -> (w8:dbl)
  n191 = Bundle(w8, w9) -> (w13:cluster{dbl, i32})  [unwired: 1 in]
  n192 = property class="Pict"(reference=w23, "Origin"=T9 {"Horizontal"=0, "Vertical"=750}, "Draw Area Size"=T8 {"Width"=624, "Height"=612}, "Position"=w13) -> ()  [unwired: 1 in, 2 out]
  n193 = Compound Arithmetic op=ADD(39.0 ("value"), w8) -> (w6:dbl)
  n194 = Bundle(w6, w9) -> (w12:cluster{dbl, i32})  [unwired: 1 in]
  n195 = property class="Pict"(reference=w20, "Draw Area Size"=T8 {"Width"=540, "Height"=540}, "Position"=w12) -> ()  [unwired: 1 in, 2 out]
  n196 = control-ref of="Camera Perf"() -> (w5:refnum<vi>)
  n197 = in-place {
    in-place-border: w18 -> [w413]
    in-place-border: [w412] -> w94
    w409 = 2.5 ("y")
    n198 = Unbundle(w413) -> ("Width"=w411:i16, "Height"=w410:i16)
    n199 = Divide(x=w410, y=w409) -> (x/y=w407:dbl)
    n200 = Divide(x=w411, y=w409) -> (x/y=w408:dbl)
    n201 = Bundle(cluster=w413, "Width"=w408, "Height"=w407) -> (w412:cluster{"Width":i16, "Height":i16})
  }
  n202 = control-ref of="Drive Base"() -> (w95:refnum<vi>)
  n203 = control-ref of="Cascade"() -> (w100:refnum<vi>)
  n204 = control-ref of="Carriage"() -> (w99:refnum<vi>)
  n205 = control-ref of="Floating"() -> (w98:refnum<vi>)
  n206 = control-ref of="Rhino"() -> (w97:refnum<vi>)
  n207 = control-ref of="Stilts"() -> (w96:refnum<vi>)
  n208 = Unbundle(w18) -> ("Width"=w90:i16)  [unwired: 1 out]
  n209 = Unbundle(w4) -> ("X"=w92:i32)  [unwired: 1 out]
  n210 = control-ref of="Endgame?"() -> (w119:refnum<vi>)
  n211 = Unbundle(w4) -> ("X"=w41:i32)  [unwired: 1 out]
  n212 = Unbundle(w18) -> ("Width"=w74:i16, "Height"=w78:i16)
  n213 = control-ref of="Postmatch Pressure Log"() -> (w102:refnum<vi>)
  n214 = Unbundle(w4) -> ("X"=w55:i32, "Y"=w52:i32)
  n215 = Unbundle(w72) -> ("Height"=w71:i16)  [unwired: 1 out]
  n216 = Unbundle(w18) -> ("Width"=w47:i16, "Height"=w44:i16)
  n217 = Divide(x=w90, y=i16 2) -> (x/y=w89:dbl)
  n218 = Divide(x=w74, y=i16 2) -> (x/y=w85:dbl)
  n219 = Compound Arithmetic op=unknown(10 ("value"), w55) -> (w53:i32)
  n220 = property class="Bool (strict)"(reference=w119, "Position"=w4, "Button Size"=w18) -> ()  [unwired: 1 in, 2 out]
  n221 = Add(x=w71, y=i16 40) -> (x+y=w2:i16)
  n222 = Divide(x=w74, y=i16 3) -> (x/y=w75:dbl)
  n223 = Divide(x=w78, y=i16 3) -> (x/y=w77:dbl)
  n224 = Build Array(w95, w100, w99, w98, w97, w96) -> (w88:refnum<vi>[])
  n225 = Compound Arithmetic op=ADD(w89, w92) -> (w93:dbl)
  n226 = Compound Arithmetic op=unknown(50 ("value"), w52) -> (w50:i32)
  n227 = Divide(x=w47, y=i16 2) -> (x/y=w45:dbl)
  n228 = Compound Arithmetic op=ADD(w41, 200.0 ("value"), w85) -> (w83:dbl)
  n229 = for {
    tunnel: w88 -> [w416] mode=indexing
    tunnel: w93 -> [w424]
    i -> [w420]
    n230 = Multiply(x=w420, y=50.0) -> (x*y=w421:dbl)
    n231 = Add(x=w421, y=100.0) -> (x+y=w419:dbl)
    n232 = Bundle(cluster=cluster{"X":i32, "Y":i32} {"X"=0, "Y"=0}, "X"=w424, "Y"=w419) -> (w418:cluster{"X":i32, "Y":i32})
    n233 = property class="Bool (strict)"(reference=w416, "Position"=w418, "Button Size"=cluster{"Width":u32, "Height":u32} {"Width"=30, "Height"=30}, "DisabledEnum"=T14."Disabled" ("Disabled")) -> ()  [unwired: 1 in, 2 out]
  }
  n234 = Bundle(cluster=w18, "Width"=w45, "Height"=w44) -> (w43:cluster{"Width":i16, "Height":i16})
  n235 = Bundle(cluster=w4, "X"=w53, "Y"=w50) -> (w49:cluster{"X":i32, "Y":i32})
  n236 = Bundle(cluster=w4, "X"=w53, "Y"=w52) -> (w56:cluster{"X":i32, "Y":i32})
  n237 = Bundle(cluster=w4, "X"=500, "Y"=w2) -> (w60:cluster{"X":i32, "Y":i32})
  n238 = Bundle(cluster=w4, "X"=i16 400 ("y"), "Y"=w2) -> (w63:cluster{"X":i32, "Y":i32})
  n239 = Bundle(cluster=w4, "X"=i16 230 ("y"), "Y"=w2) -> (w65:cluster{"X":i32, "Y":i32})
  n240 = Bundle(cluster=w4, "X"=0, "Y"=w2) -> (w69:cluster{"X":i32, "Y":i32})
  n241 = Bundle(cluster=w4, "X"=w83, "Y"=100.0) -> (w81:cluster{"X":i32, "Y":i32})
  n242 = Bundle(cluster=w18, "Width"=w75, "Height"=w77) -> (w80:cluster{"Width":i16, "Height":i16})
  n243 = property class="WFChart (strict)"(reference=w102, "Position"=w4, "Plot Area Size"=w94) -> ()  [unwired: 1 in, 2 out]
  n244 = Bundle(cluster=w4, "X"=600, "Y"=w2) -> (w3:cluster{"X":i32, "Y":i32})
  n245 = in-place {
    in-place-border: w18 -> [w434]
    in-place-border: [w433] -> w103
    in-place-border: w114 -> [w431]
    in-place-border: 1.5 ("y") -> [w428]
    in-place-border: [w426] -> w112
    in-place-border: [w425] -> w111
    n246 = Unbundle(w434) -> ("Width"=w425:i16, "Height"=w432:i16)
    n247 = Multiply(x=w431, y=i16 2) -> (x*y=w430:i16)
    n248 = Subtract(x=w432, y=w430) -> (x-y=w427:i16)
    n249 = Multiply(x=w428, y=w427) -> (x*y=w426:dbl)
    n250 = Bundle(cluster=w434, "Width"=w426, "Height"=w427) -> (w433:cluster{"Width":i16, "Height":i16})
  }
  n251 = control-ref of="Tree"() -> (w48:refnum<vi>)
  n252 = control-ref of="IMU"() -> (w58:refnum<vi>)
  n253 = control-ref of="Autonomous Selector"() -> (w57:refnum<vi>)
  n254 = control-ref of="Driver Configuration"() -> (w61:refnum<vi>)
  n255 = control-ref of="Rec Mode"() -> (w62:refnum<vi>)
  n256 = control-ref of="DB Camera Config"() -> (w66:refnum<vi>)
  n257 = control-ref of="Camera Name Right"() -> (w73:refnum<vi>)
  n258 = control-ref of="Errors"() -> (w87:refnum<vi>)
  n259 = property class="RadioBtnsControl (strict)"(reference=w62, "Position"=w63) -> ()  [unwired: 1 in, 2 out]
  n260 = property class="Str"(reference=w5, "Position"=w3) -> ()  [unwired: 1 in, 2 out]
  n261 = property class="DigNum (strict)"(reference=w58, "Position"=w49) -> ()  [unwired: 1 in, 2 out]
  n262 = property class="Enum (strict)"(reference=w57, "Position"=w56) -> ()  [unwired: 1 in, 2 out]
  n263 = property class="Enum (strict)"(reference=w61, "Position"=w60) -> ()  [unwired: 1 in, 2 out]
  n264 = property class="Bool (strict)"(reference=w66, "Position"=w65) -> ()  [unwired: 1 in, 2 out]
  n265 = property class="Tree (strict)"(reference=w48, "Position"=cluster{"Left":i32, "Top":i32} {"Left"=10, "Top"=35}, "Size"=w43) -> ()  [unwired: 1 in, 2 out]
  n266 = control-ref of="Time"() -> (w109:refnum<vi>)
  n267 = in-place {
    in-place-border: w4 -> [w447]
    in-place-border: [w446] -> w104
    in-place-border: w114 -> [w443]
    in-place-border: w112 -> [w442]
    in-place-border: w111 -> [w436]
    n268 = Unbundle(w447) -> ("X"=w440:i32, "Y"=w445:i32)
    n269 = Divide(x=w442, y=2.0) -> (x/y=w441:dbl)
    n270 = Divide(x=w436, y=2.0) -> (x/y=w435:dbl)
    n271 = Add(x=w445, y=w443) -> (x+y=w444:i32)
    n272 = Compound Arithmetic op=ADD(w440, invert w441, w435) -> (w439:dbl)
    n273 = Bundle(cluster=w447, "X"=w439, "Y"=w444) -> (w446:cluster{"X":i32, "Y":i32})
  }
  n274 = property class="CmbBox"(reference=w73, "Position"=w69) -> ()  [unwired: 1 in, 2 out]
  n275 = control-ref of="Pressure"() -> (w105:refnum<vi>)
  n276 = property class="Str"(reference=w87, "Position"=w81, "Size"=w80) -> ()  [unwired: 1 in, 2 out]
  n277 = property class="DigNum (strict)"(reference=w109) -> ("Bounds"=w108:T8)  [unwired: 1 in, 2 out]
  n278 = property class="Slide (strict)"(reference=w105) -> ("Bounds"=w107:T8)  [unwired: 1 in, 2 out]
  n279 = control-ref of="Camera Image Right"() -> (w115:refnum<vi>)
  n280 = property class="ImageControl"(reference=w115, "Position"=w104, "Image Area Size"=w103) -> ()  [unwired: 1 in, 2 out]
  n281 = in-place {
    in-place-border: w4 -> [w470]
    in-place-border: [w469] -> w110
    in-place-border: w18 -> [w466]
    in-place-border: w108 -> [w462]
    in-place-border: w104 -> [w458]
    n282 = Unbundle(w470) -> ("X"=w449:i32, "Y"=w467:i32)
    n283 = Unbundle(w466) -> ("Height"=w464:i16)  [unwired: 1 out]
    n284 = Unbundle(w458) -> ("X"=w455:i32)  [unwired: 1 out]
    n285 = Unbundle(w462) -> ("Width"=w456:u32, "Height"=w460:u32)
    n286 = Divide(x=w464, y=2.0) -> (x/y=w463:dbl)
    n287 = Compound Arithmetic op=ADD(invert w449, w455) -> (w453:i32)
    n288 = Divide(x=w460, y=2.0) -> (x/y=w459:dbl)
    n289 = Divide(x=w456, y=2.0) -> (x/y=w451:dbl)
    n290 = Divide(x=w453, y=2.0) -> (x/y=w452:dbl)
    n291 = Subtract(x=w452, y=w451) -> (x-y=w450:dbl)
    n292 = Add(x=w449, y=w450) -> (x+y=w448:dbl)
    n293 = Compound Arithmetic op=ADD(w467, invert w459, w463) -> (w468:dbl)
    n294 = Bundle(cluster=w470, "X"=w448, "Y"=w468) -> (w469:cluster{"X":i32, "Y":i32})
  }
  n295 = in-place {
    in-place-border: w4 -> [w494]
    in-place-border: [w493] -> w106
    in-place-border: w18 -> [w490]
    in-place-border: w107 -> [w486]
    in-place-border: w104 -> [w482]
    in-place-border: w103 -> [w481]
    n296 = Unbundle(w494) -> ("Y"=w491:i32)  [unwired: 1 out]
    n297 = Unbundle(w490) -> ("Width"=w478:i16, "Height"=w488:i16)
    n298 = Unbundle(w482) -> ("X"=w474:i32)  [unwired: 1 out]
    n299 = Unbundle(w481) -> ("Width"=w473:i16)  [unwired: 1 out]
    n300 = Unbundle(w486) -> ("Width"=w475:u32, "Height"=w484:u32)
    n301 = Divide(x=w488, y=2.0) -> (x/y=w487:dbl)
    n302 = Divide(x=w484, y=2.0) -> (x/y=w483:dbl)
    n303 = Divide(x=w475, y=2.0) -> (x/y=w472:dbl)
    n304 = Compound Arithmetic op=ADD(invert w474, invert w473, w478) -> (w479:i32)
    n305 = Divide(x=w479, y=2.0) -> (x/y=w477:dbl)
    n306 = Compound Arithmetic op=ADD(invert w472, w474, w473, w477) -> (w471:dbl)
    n307 = Compound Arithmetic op=ADD(w491, invert w483, w487) -> (w492:dbl)
    n308 = Bundle(cluster=w494, "X"=w471, "Y"=w492) -> (w493:cluster{"X":i32, "Y":i32})
  }
  n309 = property class="DigNum (strict)"(reference=w109, "Position"=w110) -> ()  [unwired: 1 in, 2 out]
  n310 = property class="Slide (strict)"(reference=w105, "Position"=w106) -> ()  [unwired: 1 in, 2 out]
